vi "CRYResult name channel append.vi"(10 "Curve selected":string, 11 "Limit step name (no ext.)":string) -> (3 "Result name with channel suffix":string)   [LabVIEW 2013]
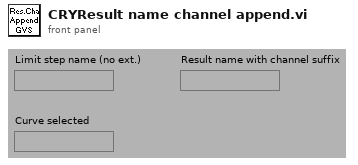
[diagram p1: front panel]
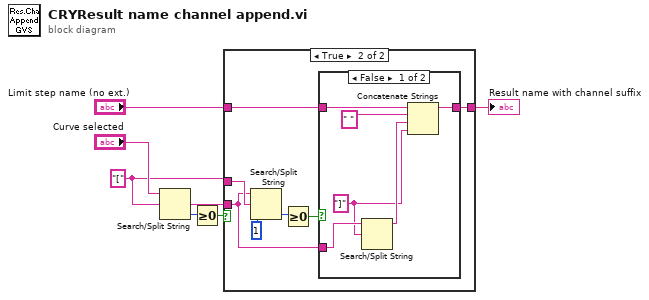
[diagram p0: block diagram]
diagram:
  w3 = "["
  n1 = Search/Split String(string="Curve selected", search string/char (-)=w3) -> (match + rest of string=w4:string, offset of match=w6:i32)  [unwired: 2 out]
  n2 = Greater Or Equal To 0?(x=w6) -> (x >= 0?=w5:bool)
  n3 = case shown="True" w5 {
    tunnel: w4 -> [_ w12]
    tunnel: w3 -> [_ w15]
    tunnel: "Limit step name (no ext.)" -> [w8 w11]
    tunnel: [w8 w10] -> w1
    frame False {
    }
    frame True {
      n4 = Search/Split String(string=w12, search string/char (-)=w15, offset (0)=1) -> (offset of match=w14:i32)  [unwired: 2 out]
      n5 = Greater Or Equal To 0?(x=w14) -> (x >= 0?=w13:bool)
      n6 = case shown="False" w13 {
        tunnel: w12 -> [w21 _]
        tunnel: w11 -> [w20 w22]
        tunnel: [w16 w22] -> w10
        frame False {
          w17 = "]"
          n7 = Search/Split String(string=w21, search string/char (-)=w17) -> (substring before match=w18:string)  [unwired: 3 out]
          n8 = Concatenate Strings(w20, " ", w18, w17) -> (w16:string)
        }
        frame True {
        }
      }
    }
  }
  "Result name with channel suffix" <- w1
